vi "draw correction factor.vi"(8 "error in (no error)":errorcluster, 11 "Path":path=path "C:/labview project/PSA SubVIs/temp file/cable.csv") -> (0 "error out":errorcluster, 1 "Factor 1D array":dbl[](array[numeric]), 2 "Stop F":dbl, 3 "Start F (MHz)":dbl)   [LabVIEW 2016]
doc: "transfer correction factor (antenna factor, cable loss, amplifier, attenuator, etc, ) from CSV file to a 1D Array, so it can be dispayed in graph."
panel:
  out "Waveform Graph":dbl[](graph)
  out "Output Array":dbl[][](array[numeric])
  out "Number of Columns":i32
  out "Number of Rows":i32
  # "(MHz)"
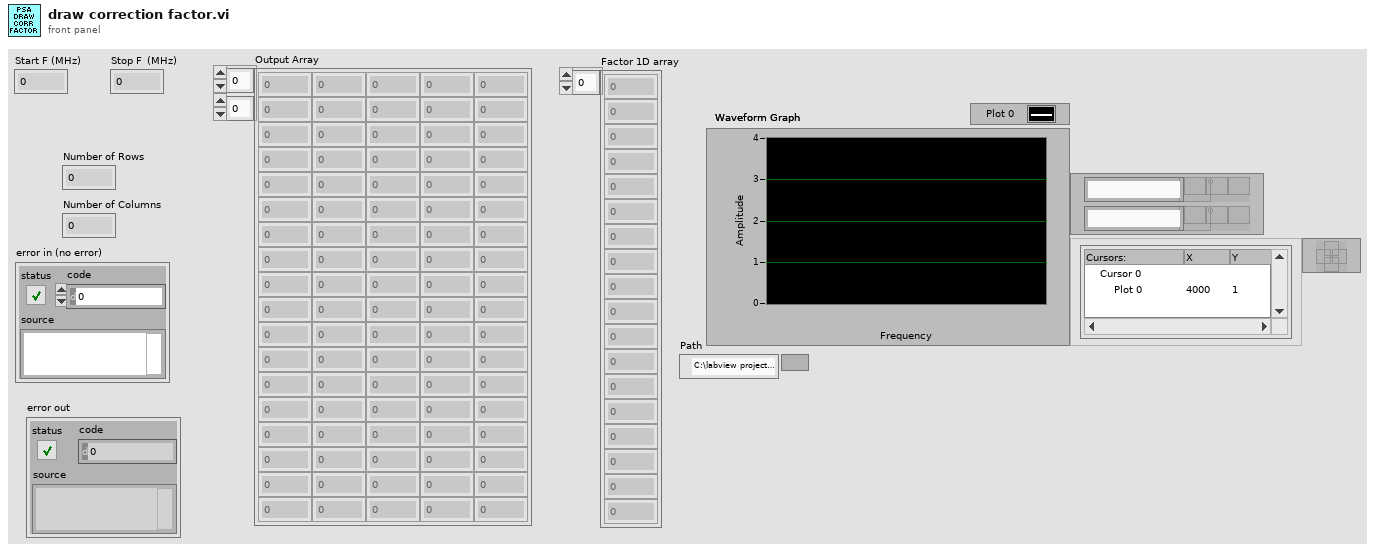
[diagram p1: front panel]
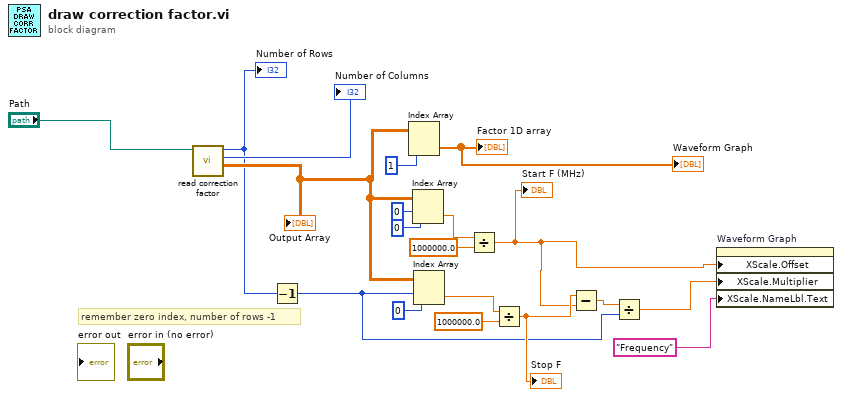
[diagram p0: block diagram]
diagram:
  # "remember zero index, number of rows -1"
  n1 = call "read correction factor.vi"("Path"="Path") -> ("Output Array"=w15:dbl[][], "Number of Columns"=→"Number of Columns":i32, "Number of Rows"=w5:i32)  [unwired: 7 in, 1 out]
  "Number of Rows" <- w5
  "Output Array" <- w15
  n2 = Decrement(x=w5) -> (x-1=w4:i32)
  n3 = Index Array(array=w15, index (col)=1 ("disabled index (col)")) -> (element=→"Factor 1D array" →"Waveform Graph":dbl[])  [unwired: 1 in]
  n4 = Index Array(array=w15, index (row)=0, index (col)=0 ("disabled index (col)")) -> (element=w12:dbl)
  n5 = Index Array(array=w15, index (row)=w4, index (col)=0 ("disabled index (col)")) -> (element=w8:dbl)
  n6 = Divide(x=w12, y=1000000.0) -> (x/y=w3:dbl)
  "Start F (MHz)" <- w3
  n7 = Divide(x=w8, y=1000000.0) -> (x/y=w7:dbl)
  "Stop F" <- w7
  n8 = Subtract(x=w7, y=w3) -> (x-y=w13:dbl)
  n9 = Divide(x=w13, y=w4) -> (x/y=w2:dbl)
  n10 = property on="Waveform Graph" class="WFGraph (strict)"("XScale.Offset"=w3, "XScale.Multiplier"=w2, "XScale.NameLbl.Text"="Frequency" ("X Scale.Unit Label.Text")) -> ()  [unwired: 2 in, 2 out]
